vi "EIP PLC Info.vi"(5 "Message Type":T1, 6 "Path":string, 7 "Timeout":i32) -> (1 "Device Settings":T2)   [LabVIEW 2023, in "Ethernet IP Custom Device Custom Device.lvlib"]
doc: "VI that creates a cluster including the timeout when communicating with Ethernet/IP + the actual network path to the PLC."
uses:
  Ethernet IP Custom Device Custom Device.lvlib
  EIP Device Settings.ctl
  EIP Message Type.ctl
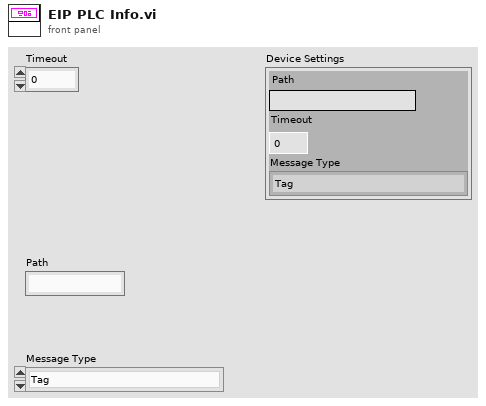
[diagram p1: front panel]
types:
  T1 = typedef "Ethernet IP Custom Device Custom Device.lvlib/EIP Message Type.ctl" = enum16{"Tag", "Assembly"}
  T2 = typedef "Ethernet IP Custom Device Custom Device.lvlib/EIP Device Settings.ctl" = cluster{"Path":string, "Timeout":i32, "Message Type":T1}
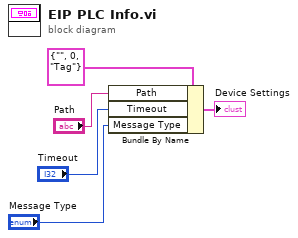
[diagram p0: block diagram]
diagram:
  n1 = Bundle By Name(cluster=T2 {"Path"="", "Timeout"=0, "Message Type"=enum."Tag"} ("Device Settings"), "Path"="Path", "Timeout"="Timeout", "Message Type"="Message Type") -> (→"Device Settings":T2)
